vi "SUB_COM_W_CharByChar.vi"(2 "cmd string":string, 3 "duplicate VISA resource name":refnum<visa-resource-name>) -> (1 "VISA resource OUT":refnum<visa-resource-name>)   [LabVIEW 2011]
panel:
  out "out1":string
  out "LOOP":i32
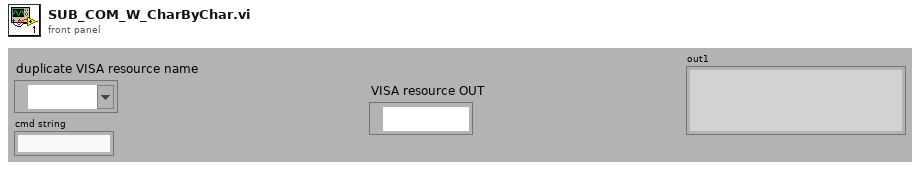
[diagram p1: front panel]
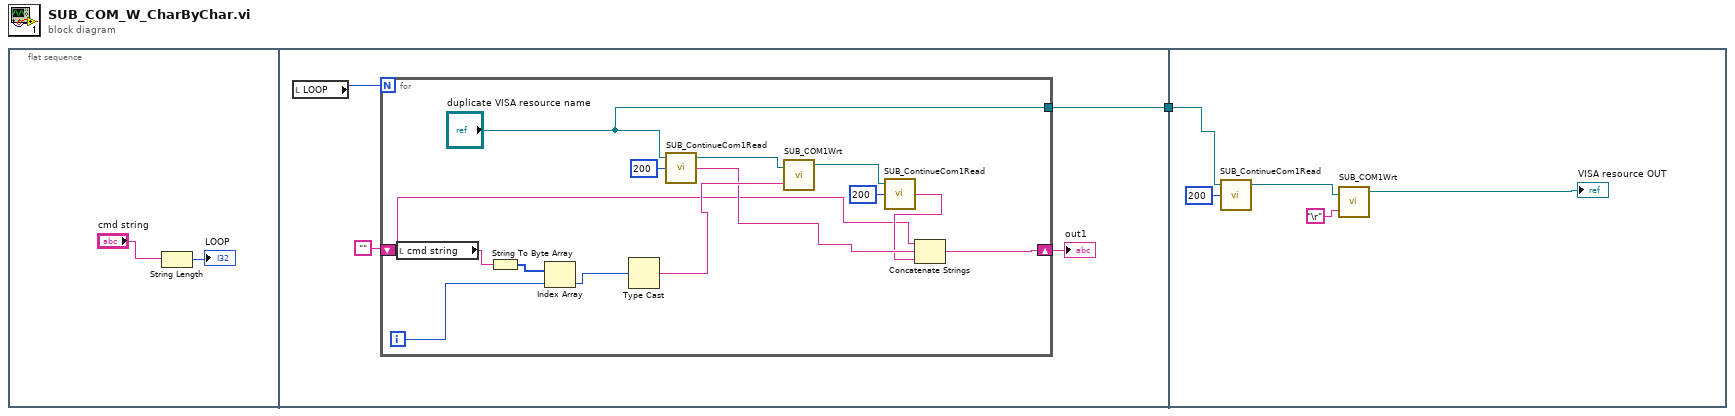
[diagram p0: block diagram]
diagram:
  n1 = flat-sequence {
    tunnel: [w6] -> w1
    tunnel: w1 -> [w24]
    frame #0 {
      n2 = String Length(string="cmd string") -> (length=→"LOOP":i32)
    }
    frame #1 {
      n3 = local read "LOOP"() -> (w7:i32)
      n4 = for {
        N: w7 -> [_]
        tunnel: ["duplicate VISA resource name"] -> w6
        shift-right: [w9] -> w4
        shift-left: "" -> [w8]
        i -> [w15]
        n5 = local read "cmd string"() -> (w17:string)
        n6 = String To Byte Array(string=w17) -> (unsigned byte array=w16:u8[])
        n7 = Index Array(array=w16, index=w15) -> (element=w14:u8)
        n8 = Type Cast(x=w14) -> (*(type *) &x=w13:string)  [unwired: 1 in]
        n9 = call "SUB_ContinueCom1Read.vi"("Numeric"=200, "duplicate VISA resource name 2"="duplicate VISA resource name") -> ("String"=w11:string, "duplicate VISA resource name"=w18:refnum<visa-resource-name>)  [unwired: 1 in, 1 out]
        n10 = call "SUB_COM1Wrt.vi"("VISA resource name"=w18, "write buffer"=w13) -> ("duplicate VISA resource name"=w20:refnum<visa-resource-name>)  [unwired: 2 out]
        n11 = call "SUB_ContinueCom1Read.vi"("Numeric"=200, "duplicate VISA resource name 2"=w20) -> ("String"=w10:string)  [unwired: 1 in, 2 out]
        n12 = Concatenate Strings(w8, w11, w10) -> (w9:string)
      }
      "out1" <- w4
    }
    frame #2 {
      n13 = call "SUB_ContinueCom1Read.vi"("Numeric"=200, "duplicate VISA resource name 2"=w24) -> ("duplicate VISA resource name"=w25:refnum<visa-resource-name>)  [unwired: 1 in, 2 out]
      n14 = call "SUB_COM1Wrt.vi"("VISA resource name"=w25, "write buffer"="\r") -> ("duplicate VISA resource name"=→"VISA resource OUT":refnum<visa-resource-name>)  [unwired: 2 out]
    }
  }
